vi "Ramps (SubVI).vi"(11 "canExecute?":bool) -> ()   [LabVIEW 2017]
uses:
  Control 1.ctl
panel:
  in  "Button2 Pushed?":bool
  in  "Button1 Pushed?":bool
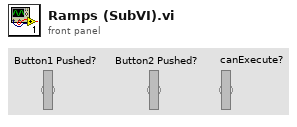
[diagram p1: front panel]
types:
  T1 = typedef "Control 1.ctl" = enum16{"folded", "expanded"}
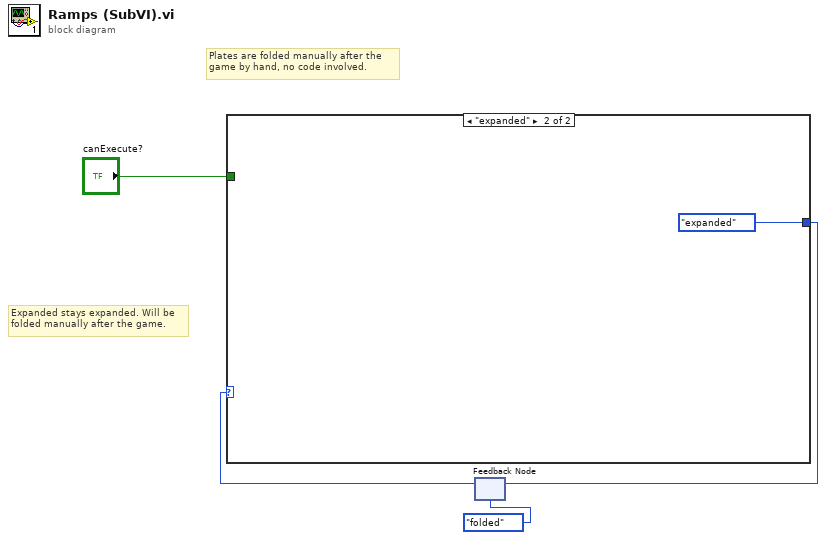
[diagram p0: block diagram]
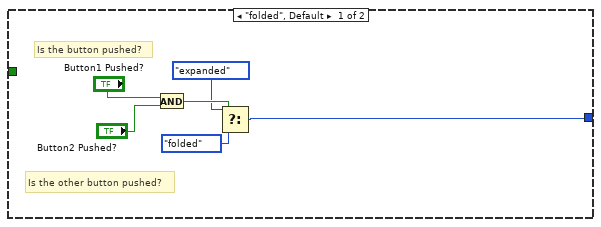
[diagram p2: hidden frame]
diagram:
  # "Expanded stays expanded. Will be\nfolded manually after the game."
  # "Plates are folded manually after the \ngame by hand, no code involved."
  n1 = feedback #1(Control_1."folded") -> (w2:T1)
  n2 = case shown="\"expanded\"" w2 {
    tunnel: [w5 Control_1."expanded"] -> w3
    tunnel: "canExecute?" -> [_ _]
    frame "folded", Default {
      # "Is the other button pushed?"
      # "Is the button pushed?"
      n3 = And(x="Button1 Pushed?", y="Button2 Pushed?") -> (x .and. y?=w8:bool)
      n4 = Select(t=Control_1."expanded", s=w8, f=Control_1."folded") -> (s? t:f=w5:T1)
    }
    frame "expanded" {
    }
  }
  n5 = feedback-in #1(w3) -> ()
